vi "Game Slide.vi"(7 "Numeric in":i32) -> (2 "Game Slide":dbl, 8 "Step":dbl)   [LabVIEW 2010]
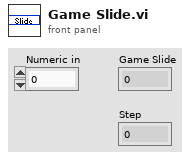
[diagram p1: front panel]
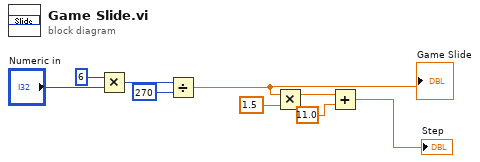
[diagram p0: block diagram]
diagram:
  n1 = Multiply(x=6, y="Numeric in") -> (x*y=w3:i32)
  n2 = Divide(x=w3, y=270) -> (x/y=w6:dbl)
  "Game Slide" <- w6
  n3 = Multiply(x=w6, y=1.5) -> (x*y=w8:dbl)
  n4 = Add(x=w8, y=11.0) -> (x+y=→"Step":dbl)
